vi "_RT Read XML MR Param.vi"(4 "error in":errorcluster, 7 "XML String":string) -> (0 "error out":errorcluster, 1 "Parameters":T1[](array[typedef]), 3 "Remaining String":string)   [LabVIEW 2015]
uses:
  Type/_Mass Range Parameters.ctl
  Type/_XML Type.ctl
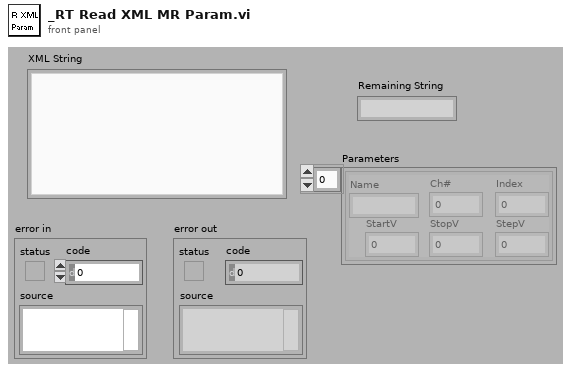
[diagram p1: front panel]
types:
  T1 = typedef "_Mass Range Parameters.ctl" = cluster{"Name":string, "Ch#":u8, "StartV":dbl, "StopV":dbl, "StepV":dbl, "Index":u8}
  T2 = typedef "_XML Type.ctl" = enum16{"Configuration", "ConTable", "Method", "Experiment", "Mass Range", "Table", "LensTable", "ParamTable", "TuneParam", "MetParam", "MassRange", "LCMethod", "LCMethodFile", "RackType", "Vial", "PlatePos", "InjVol"}
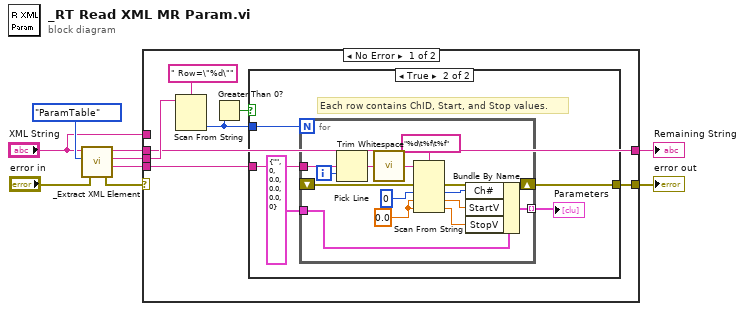
[diagram p0: block diagram]
diagram:
  n1 = call "_Extract XML Element.vi"("error in"="error in", "XML Type"=_XML_Type."ParamTable", "XML String"="XML String") -> ("error out"=w1:errorcluster, "Element"=w7:string, "Attributes"=w6:string, "Remaining String"=w5:string)  [unwired: 1 out]
  n2 = case shown="No Error" w1 {
    selector: w1 -> [_ w37]
    tunnel: [w13 w37] -> w9
    tunnel: w7 -> [w14 _]
    tunnel: w6 -> [w15 _]
    tunnel: w5 -> [w12 _]
    tunnel: "XML String" -> [_ w36]
    tunnel: [w12 w36] -> w3
    frame No Error {
      n3 = Scan From String(format string=" Row=\"%d\"", input string=w15) -> (output 1=w10:i32)  [unwired: 2 in, 4 out]
      n4 = Greater Than 0?(x=w10) -> (x > 0?=w11:bool)
      n5 = case shown="True" w11 {
        tunnel: w10 -> [_ w21]
        tunnel: w14 -> [_ w20]
        tunnel: [_ w19] -> w13
        frame False {
        }
        frame True {
          # "Each row contains ChID, Start, and Stop values."
          n6 = for {
            N: w21 -> [_]
            tunnel: w20 -> [w33]
            shift-right: [w30] -> w19
            shift-left: _ -> [w29]
            tunnel: [w25] -> w18 mode=indexing
            tunnel: T1 {"Name"="", "Ch#"=0, "StartV"=0.0, "StopV"=0.0, "StepV"=0.0, "Index"=0} ("MR Parameters") -> [w26]
            i -> [w32]
            w27 = 0.0 ("Ch#")
            n7 = Pick Line(multi-line string=w33, line index=w32) -> (output string=w34:string)  [unwired: 1 out]
            n8 = call <vilib>:"Trim Whitespace.vi"("string"=w34) -> ("trimmed string"=w31:string)  [unwired: 1 in]
            n9 = Scan From String(format string="%d\t%f\t%f", input string=w31, error in=w29, default 1=u8 0 ("Ch#"), default 2=w27, default 3=w27) -> (error out=w30:errorcluster, output 1=w24:u8, output 2=w23:dbl, output 3=w22:dbl)  [unwired: 1 in, 2 out]
            n10 = Bundle By Name(cluster=w26, "Ch#"=w24, "StartV"=w23, "StopV"=w22) -> (w25:T1)
          }
          "Parameters" <- w18
        }
      }
    }
    frame Error {
    }
  }
  "error out" <- w9
  "Remaining String" <- w3
